vi "LKIF_GetFigureData.vi"(8 "error in (no error)":errorcluster {"code" format="%x"}, 11 "OutNo (0: OUT1)":i32) -> (0 "error out":errorcluster {"code" format="%x"}, 3 "FigureData":T1 {"SdValue"."LKIF_FLOATRESULT" items=["VALID", "RANGEOVER_P", "RANGEOVER_N", "WAITING"]; "DifValue"."LKIF_FLOATRESULT" items=["VALID", "RANGEOVER_P", "RANGEOVER_N", "WAITING"]; "MinValue"."LKIF_FLOATRESULT" items=["VALID", "RANGEOVER_P", "RANGEOVER_N", "WAITING"]; "MaxValue"."LKIF_FLOATRESULT" items=["VALID", "RANGEOVER_P", "RANGEOVER_N", "WAITING"]; "AverageValue"."LKIF_FLOATRESULT" items=["VALID", "RANGEOVER_P", "RANGEOVER_N", "WAITING"]; "ToleLower"."LKIF_FLOATRESULT" items=["VALID", "RANGEOVER_P", "RANGEOVER_N", "WAITING"]; "ToleUpper"."LKIF_FLOATRESULT" items=["VALID", "RANGEOVER_P", "RANGEOVER_N", "WAITING"]})   [LabVIEW 2024, in "Keyence LK-G3000.lvlib"]
uses:
  Keyence LK-G3000.lvlib
  clusters/LKIF_FIGUREDATA.ctl
  clusters/LKIF_FLOATVALUE.ctl
  enums/LKIF_FLOATRESULT.ctl
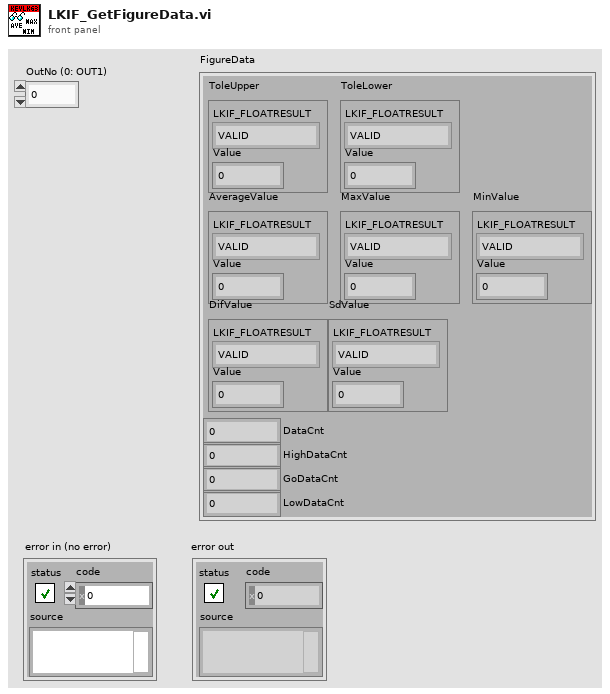
[diagram p1: front panel]
types:
  T1 = typedef "Keyence LK-G3000.lvlib/LKIF_FIGUREDATA.ctl" = cluster{"ToleUpper":T2, "ToleLower":T2, "AverageValue":T2, "MaxValue":T2, "MinValue":T2, "DifValue":T2, "SdValue":T2, "DataCnt":i32, "HighDataCnt":i32, "GoDataCnt":i32, "LowDataCnt":i32}
  T2 = typedef "Keyence LK-G3000.lvlib/LKIF_FLOATVALUE.ctl" = cluster{"LKIF_FLOATRESULT":T3, "Value":sgl}
  T3 = typedef "Keyence LK-G3000.lvlib/LKIF_FLOATRESULT.ctl" = i32
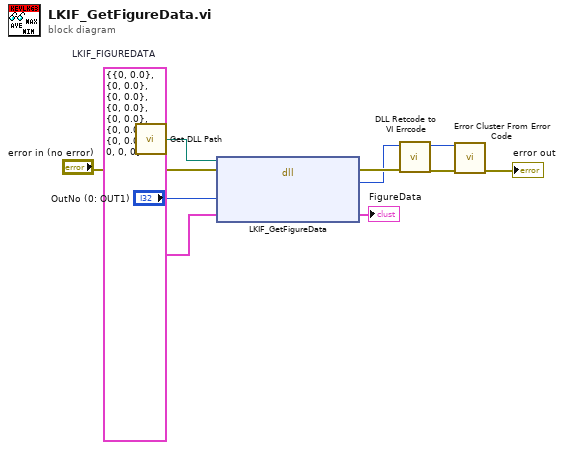
[diagram p0: block diagram]
diagram:
  w2 = T1 {"ToleUpper"={"LKIF_FLOATRESULT"=0, "Value"=0.0}, "ToleLower"={"LKIF_FLOATRESULT"=0, "Value"=0.0}, "AverageValue"={"LKIF_FLOATRESULT"=0, "Value"=0.0}, "MaxValue"={"LKIF_FLOATRESULT"=0, "Value"=0.0}, "MinValue"={"LKIF_FLOATRESULT"=0, "Value"=0.0}, "DifValue"={"LKIF_FLOATRESULT"=0, "Value"=0.0}, "SdValue"={"LKIF_FLOATRESULT"=0, "Value"=0.0}, "DataCnt"=0, "HighDataCnt"=0, "GoDataCnt"=0, "LowDataCnt"=0}  # LKIF_FIGUREDATA
  n1 = call "Get DLL Path.vi"() -> ("DLL Path"=w6:path)  [unwired: 1 in]
  n2 = dll-call lib="C:/Program Files/National Instruments/LabVIEW 2011/instr.lib/Keyence LK-G3000/LkIF.dll" fn="LKIF_GetFigureData"(path in=w6, error in="error in (no error)", "OutNo"="OutNo (0: OUT1)", "FigureData"=w2) -> (error out=w8:errorcluster, "RC"=w7:i32, "FigureData"=→"FigureData":T1)  [unwired: 2 in, 1 out]
  n3 = call "DLL Retcode to VI Errcode.vi"("error in (no error)"=w8, "DLL Retcode"=w7) -> ("error out"=w10:errorcluster, "VI Errcode"=w9:i32)  [unwired: 8 in]
  n4 = call <vilib>:"Error Cluster From Error Code.vi"("error in (no error)"=w10, "error code (0)"=w9) -> ("error out"=→"error out":errorcluster)  [unwired: 7 in]
